vi "Write Measurement Interface.vi"(8 "error in (no error)":errorcluster, 10 "Measurement Interface.lvlibp:Measurement Interface":refnum<class "Measurement Interface.lvclass">, 11 "niRFSTS Sequence Flow in":refnum<class "niRFSTS Sequence Flow.lvclass">) -> (0 "error out":errorcluster, 3 "niRFSTS Sequence Flow out":refnum<class "niRFSTS Sequence Flow.lvclass">)   [LabVIEW 2018, in "niRFSTS Sequence Flow.lvclass"]
uses:
  niRFSTS Sequence Flow.lvclass
  Plugins/Measurement Interface.lvlibp/Measurement Interface.lvclass
  niRFSTS Sequence Flow.lvclass/niRFSTS Sequence Flow.ctl
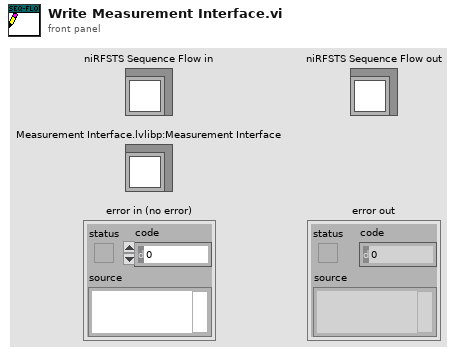
[diagram p1: front panel]
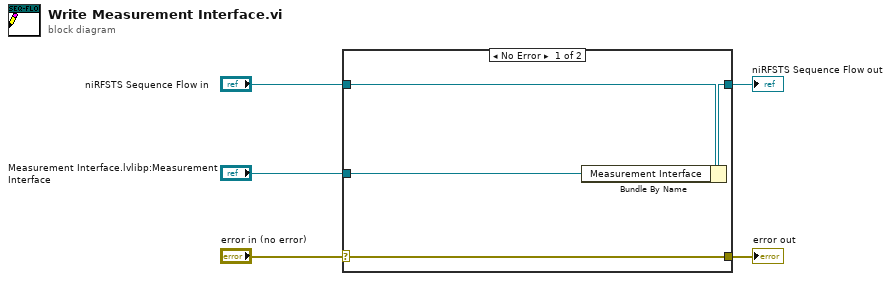
[diagram p0: block diagram]
diagram:
  n1 = case shown="No Error" "error in (no error)" {
    selector: "error in (no error)" -> [w9 w10]
    tunnel: [w9 w10] -> w4
    tunnel: [w7 w11] -> w2
    tunnel: "niRFSTS Sequence Flow in" -> [w8 w11]
    tunnel: "Measurement Interface.lvlibp:Measurement Interface" -> [w6 _]
    frame No Error {
      n2 = Bundle By Name(cluster=w8, "Measurement Interface"=w6) -> (w7:refnum<class "niRFSTS Sequence Flow.lvclass">)
    }
    frame Error {
    }
  }
  "error out" <- w4
  "niRFSTS Sequence Flow out" <- w2
